vi "Priority system.vi"(0 "robot location":dbl[](array[numeric]), 1 "robot direction":string, 2 "Target distance":dbl, 3 "Display Map":dbl[][](array[numeric])) -> (7 "Map":u16[][](array[ring]), 8 "target location":dbl[](array[numeric]))   [LabVIEW 2015]
uses:
  <vilib>/robotics/Navigation/shared/WorldMap/OccupancyGridWorldMap/NI_Robotics_OccupancyGridWorldMap.lvclass
  <vilib>/robotics/Navigation/NI_Robotics_Navigation .lvlib
panel:
  out "route map":dbl[][](array[numeric])
  out "distances":dbl[](array[numeric])
  out "Indices":i32[][](array[numeric])
  out "Priority level array":dbl[][](array[numeric])
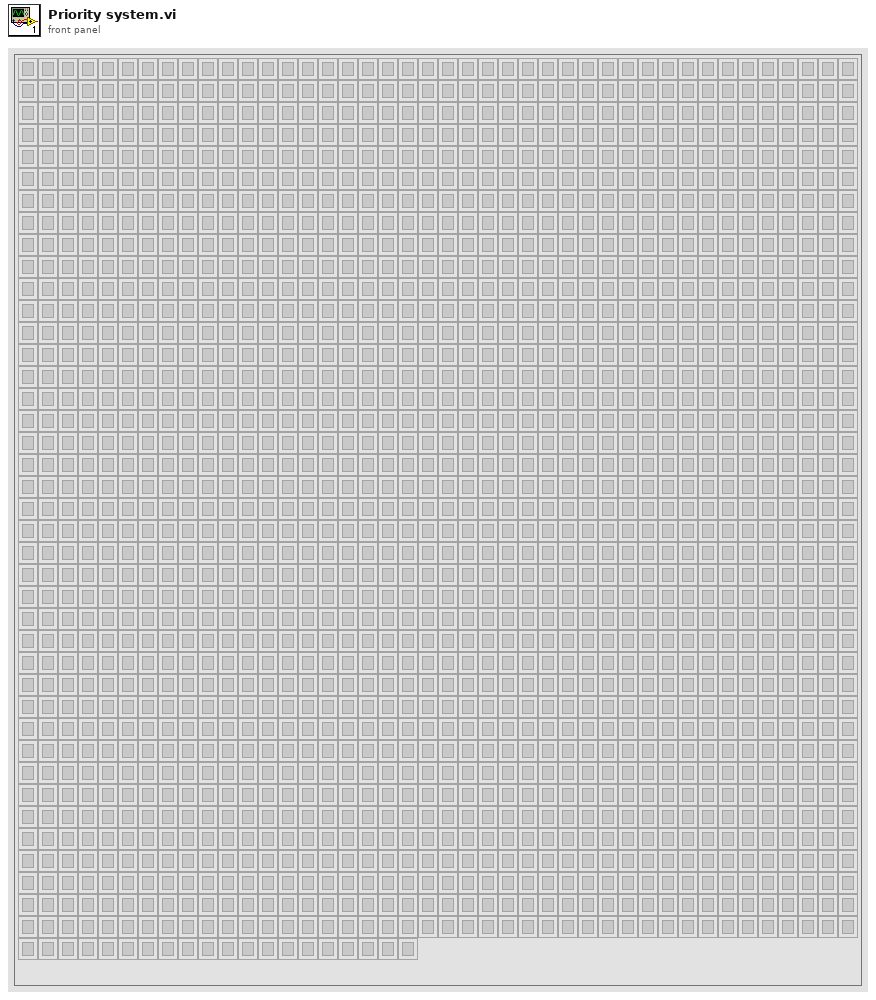
[diagram p1: front panel]
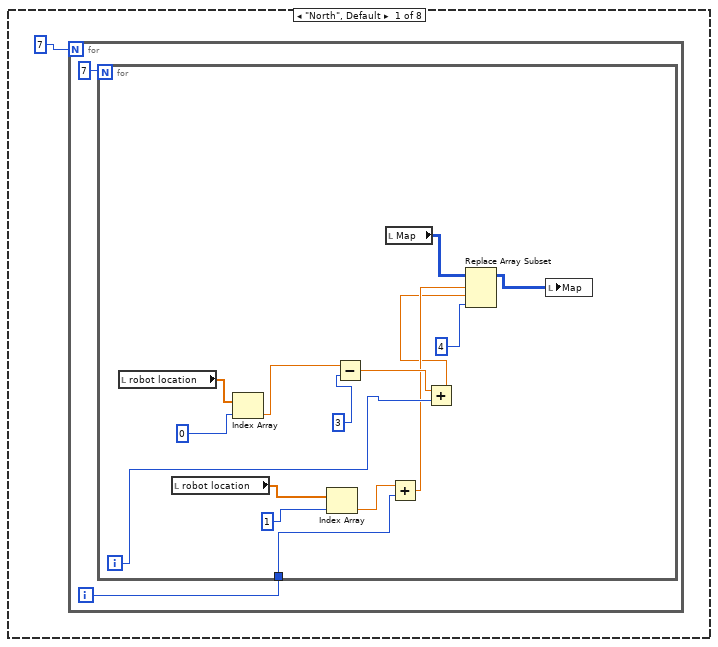
[diagram p2: hidden frame]
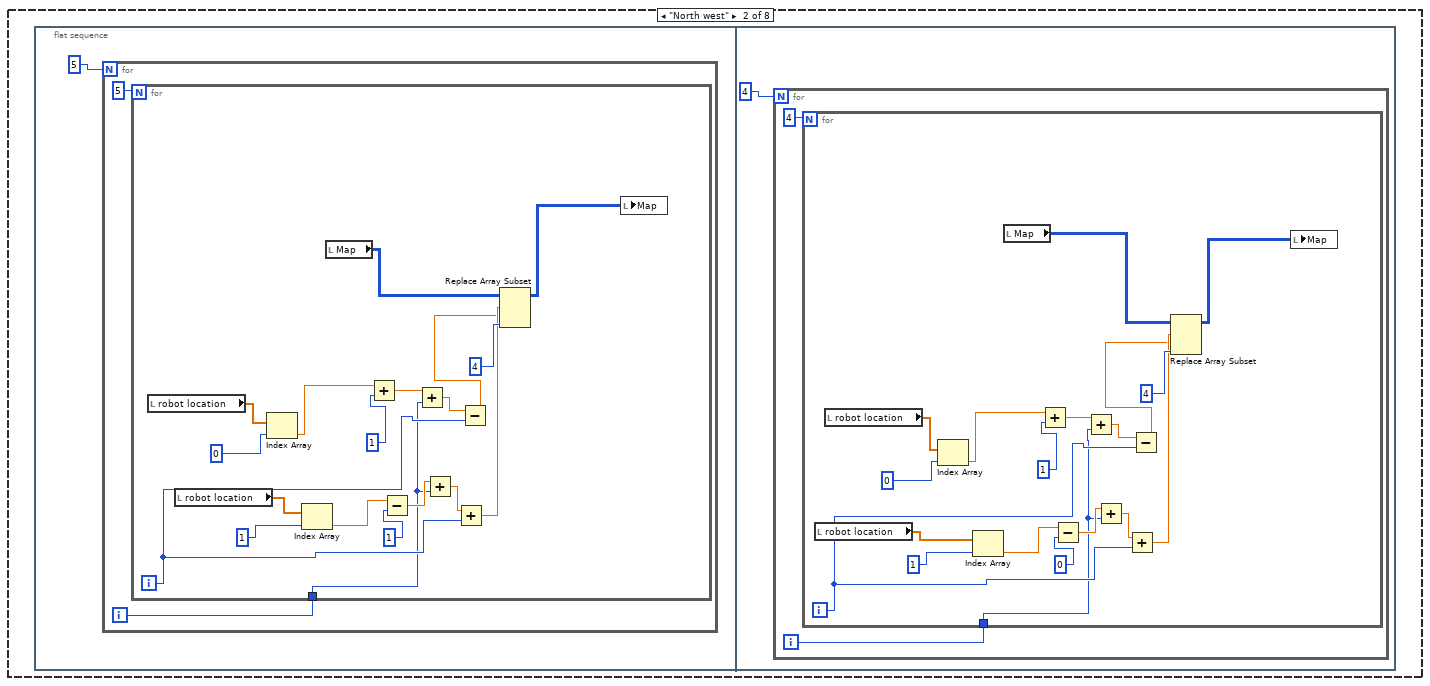
[diagram p3: hidden frame]
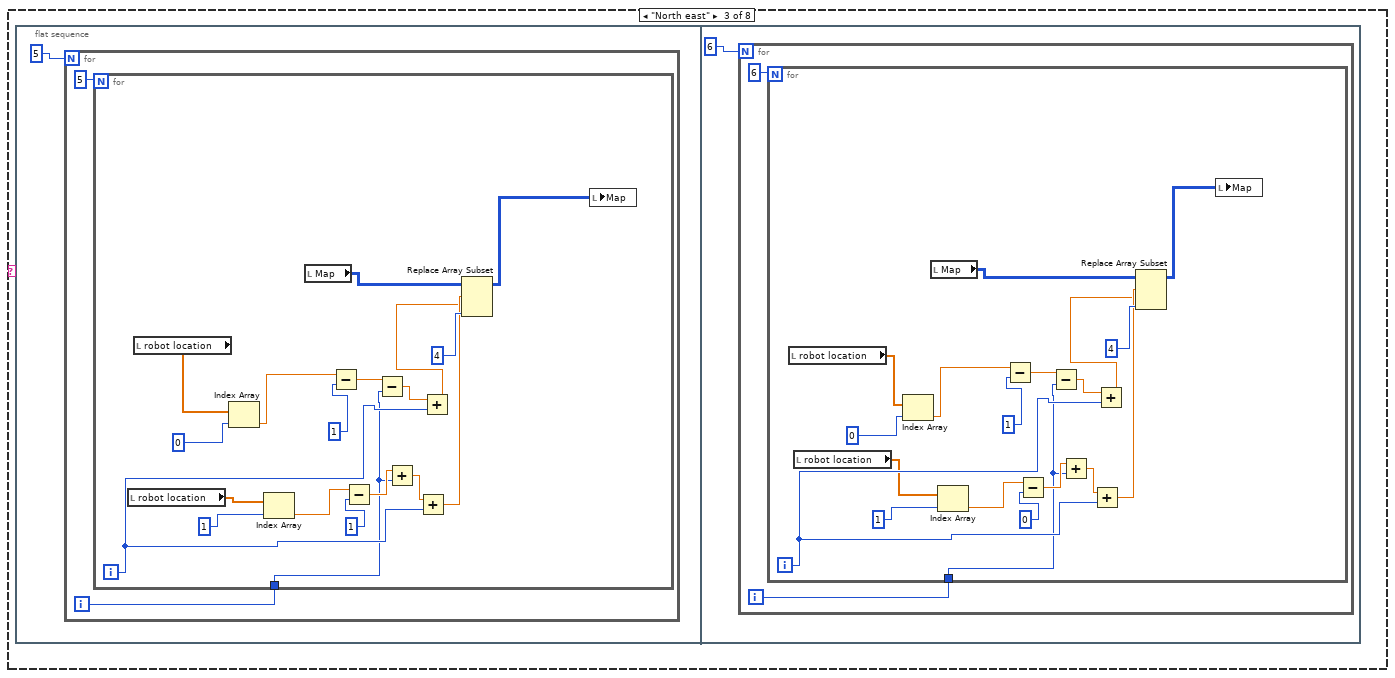
[diagram p4: hidden frame]
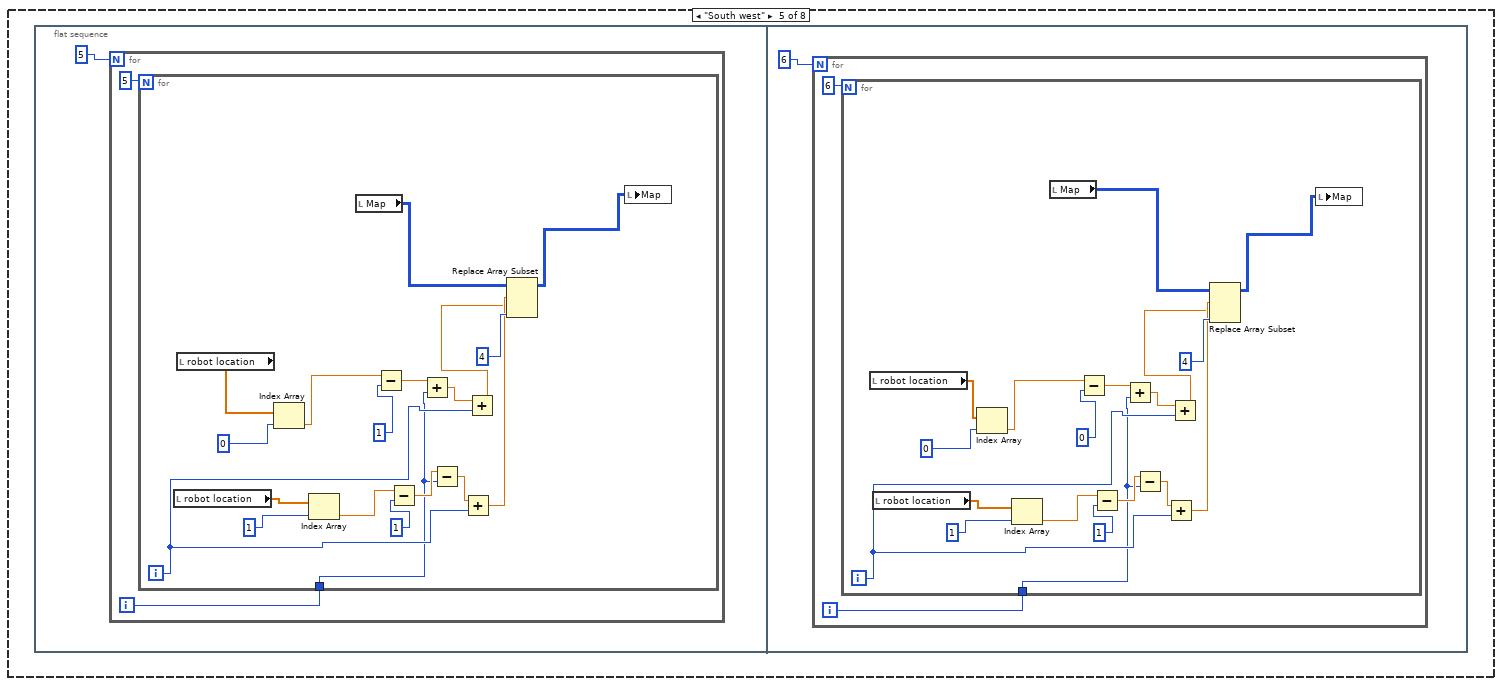
[diagram p5: hidden frame]
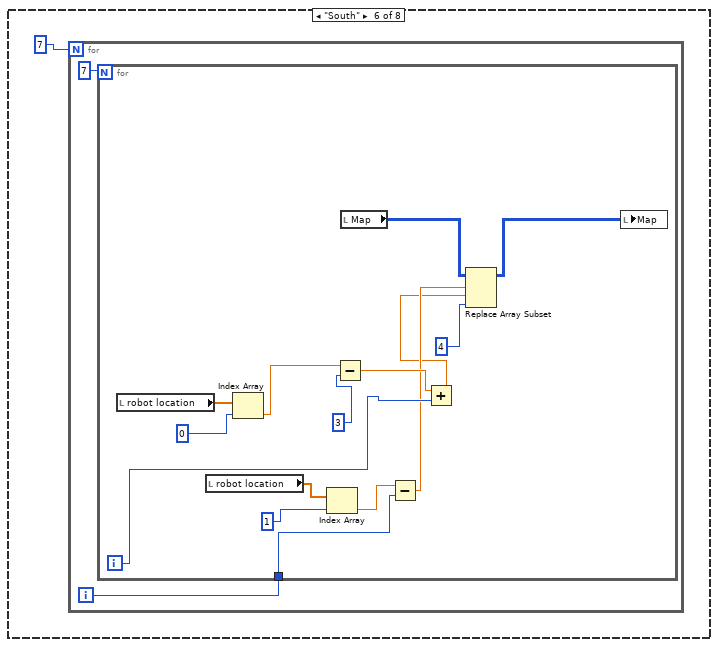
[diagram p6: hidden frame]
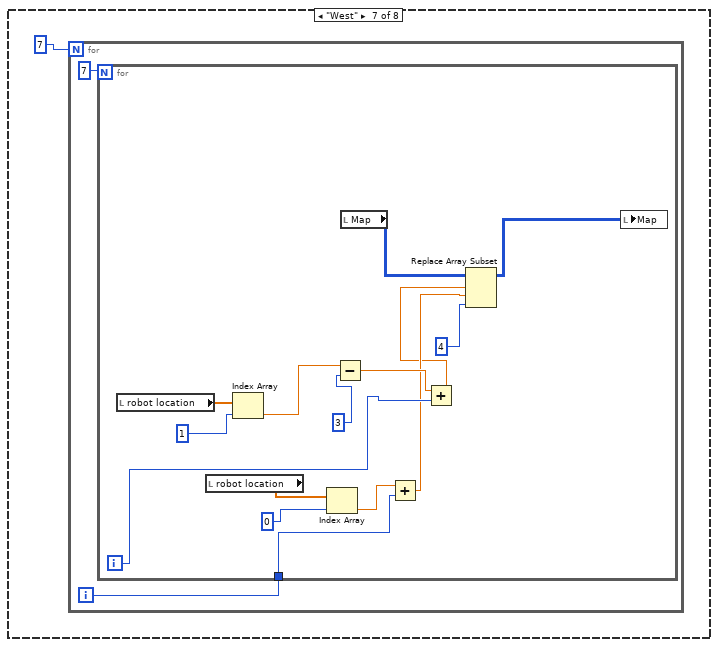
[diagram p7: hidden frame]
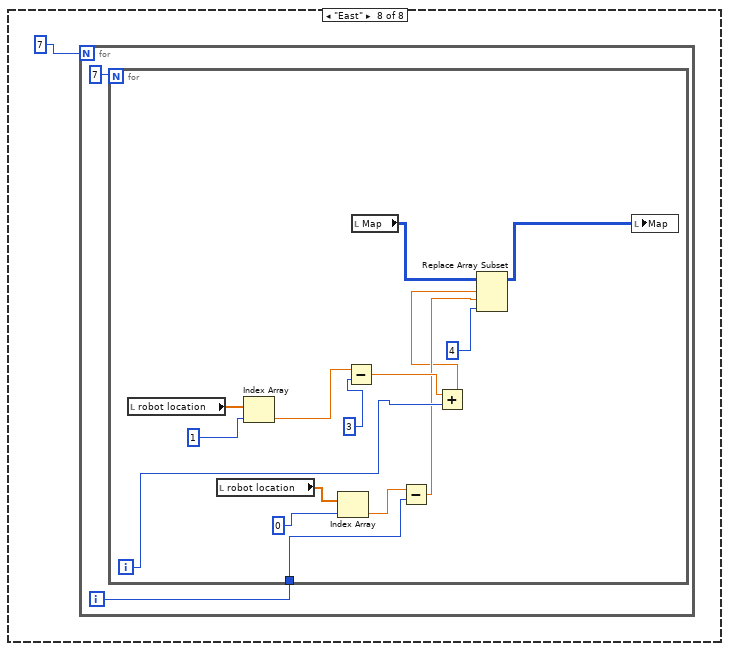
[diagram p8: hidden frame]
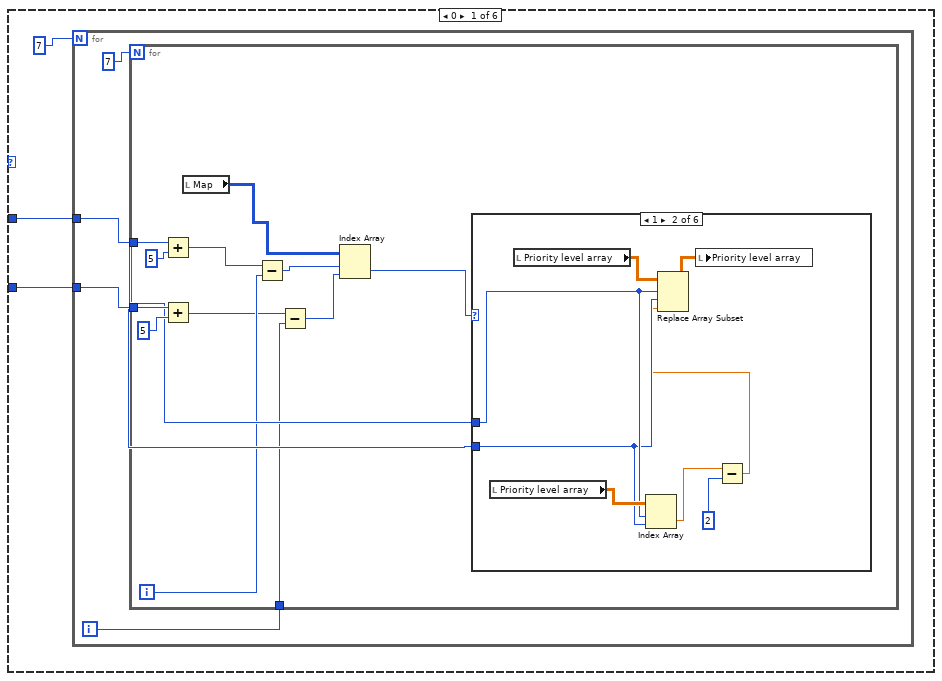
[diagram p9: hidden frame]
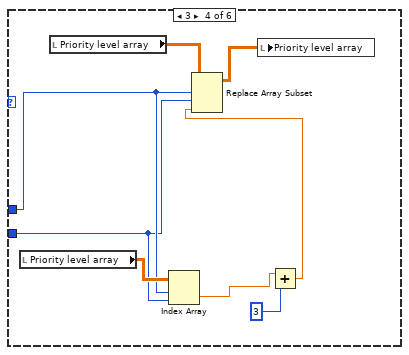
[diagram p12: hidden frame]
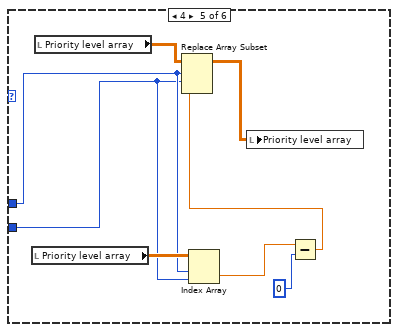
[diagram p13: hidden frame]
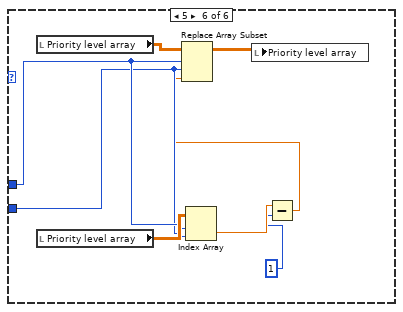
[diagram p14: hidden frame]
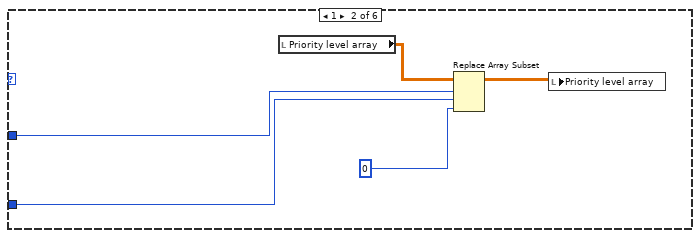
[diagram p15: hidden frame]
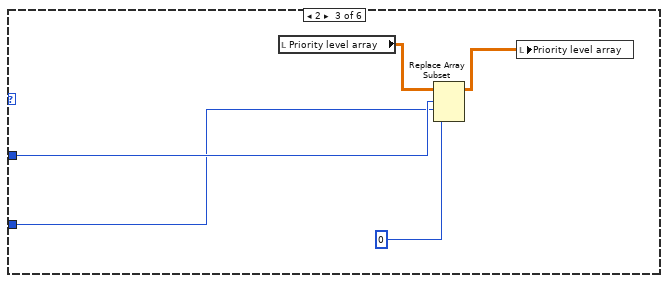
[diagram p16: hidden frame]
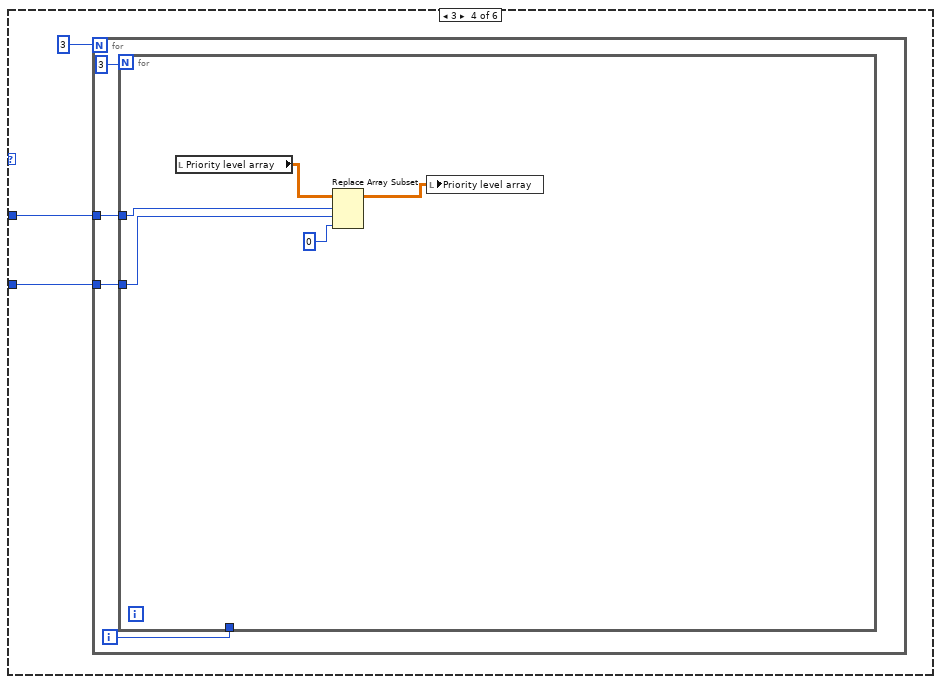
[diagram p17: hidden frame]
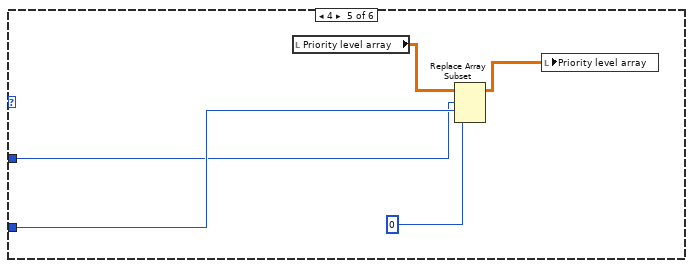
[diagram p18: hidden frame]
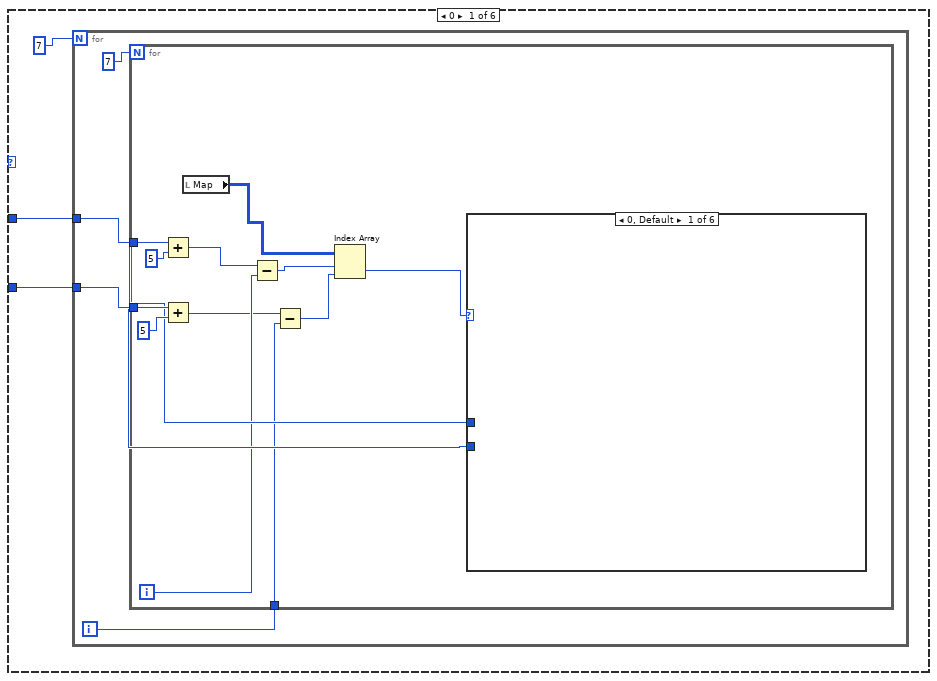
[diagram p20: hidden frame]
diagram:
  n1 = flat-sequence {
    frame #0 {
      "Map" <- "Display Map"
      "Priority level array" <- "Display Map"
      "route map" <- "Display Map"
    }
    frame #1 {
      n2 = for {
        N: 40 -> [_]
        i -> [w3]
        n3 = for {
          N: 40 -> [_]
          tunnel: w3 -> [w9]
          i -> [w10]
          n4 = local read "Priority level array"() -> (w5:dbl[][])
          n5 = local read "route map"() -> (w6:dbl[][])
          n6 = Replace Array Subset(array=w6, new element=0, index (row)=w10, index (col)=w9) -> (w11:dbl[][])
          n7 = Replace Array Subset(array=w5, new element=15, index (row)=w10, index (col)=w9) -> (w12:dbl[][])
          n8 = local write "Priority level array"(w12) -> ()
          n9 = local write "route map"(w11) -> ()
        }
      }
    }
    frame #2 {
      n10 = case shown="\"South east\"" "robot direction" {
        frame "North", Default {
          n11 = for {
            N: 7 -> [_]
            i -> [w15]
            n12 = for {
              N: 7 -> [_]
              tunnel: w15 -> [w23]
              i -> [w27]
              n13 = local read "robot location"() -> (w18:dbl[])
              n14 = local read "robot location"() -> (w17:dbl[])
              n15 = Index Array(array=w18, index=0) -> (element=w20:dbl)
              n16 = Index Array(array=w17, index=1) -> (element=w19:dbl)
              n17 = Subtract(x=w20, y=3) -> (x-y=w26:dbl)
              n18 = local read "Map"() -> (w22:u16[][])
              n19 = Add(x=w19, y=w23) -> (x+y=w25:dbl)
              n20 = Add(x=w26, y=w27) -> (x+y=w24:dbl)
              n21 = Replace Array Subset(array=w22, new element=4, index (row)=w25, index (col)=w24) -> (w21:u16[][])
              n22 = local write "Map"(w21) -> ()
            }
          }
        }
        frame "North west" {
          n23 = flat-sequence {
            frame #0 {
              n24 = for {
                N: 5 -> [_]
                i -> [w33]
                n25 = for {
                  N: 5 -> [_]
                  tunnel: w33 -> [w35]
                  i -> [w46]
                  n26 = local read "robot location"() -> (w41:dbl[])
                  n27 = local read "robot location"() -> (w40:dbl[])
                  n28 = Index Array(array=w41, index=0) -> (element=w47:dbl)
                  n29 = Index Array(array=w40, index=1) -> (element=w45:dbl)
                  n30 = local read "Map"() -> (w39:u16[][])
                  n31 = Add(x=w47, y=1) -> (x+y=w37:dbl)
                  n32 = Subtract(x=w45, y=1) -> (x-y=w43:dbl)
                  n33 = Add(x=w37, y=w35) -> (x+y=w36:dbl)
                  n34 = Add(x=w43, y=w35) -> (x+y=w42:dbl)
                  n35 = Add(x=w42, y=w46) -> (x+y=w49:dbl)
                  n36 = Subtract(x=w36, y=w46) -> (x-y=w48:dbl)
                  n37 = Replace Array Subset(array=w39, new element=4, index (row)=w49, index (col)=w48) -> (w38:u16[][])
                  n38 = local write "Map"(w38) -> ()
                }
              }
            }
            frame #1 {
              n39 = for {
                N: 4 -> [_]
                i -> [w55]
                n40 = for {
                  N: 4 -> [_]
                  tunnel: w55 -> [w62]
                  i -> [w68]
                  n41 = local read "robot location"() -> (w57:dbl[])
                  n42 = local read "robot location"() -> (w58:dbl[])
                  n43 = Index Array(array=w58, index=0) -> (element=w69:dbl)
                  n44 = Index Array(array=w57, index=1) -> (element=w67:dbl)
                  n45 = local read "Map"() -> (w60:u16[][])
                  n46 = Add(x=w69, y=1) -> (x+y=w65:dbl)
                  n47 = Subtract(x=w67, y=0) -> (x-y=w64:dbl)
                  n48 = Add(x=w65, y=w62) -> (x+y=w63:dbl)
                  n49 = Add(x=w64, y=w62) -> (x+y=w61:dbl)
                  n50 = Add(x=w61, y=w68) -> (x+y=w71:dbl)
                  n51 = Subtract(x=w63, y=w68) -> (x-y=w70:dbl)
                  n52 = Replace Array Subset(array=w60, new element=4, index (row)=w71, index (col)=w70) -> (w59:u16[][])
                  n53 = local write "Map"(w59) -> ()
                }
              }
            }
          }
        }
        frame "North east" {
          n54 = flat-sequence {
            frame #0 {
              n55 = for {
                N: 5 -> [_]
                i -> [w77]
                n56 = for {
                  N: 5 -> [_]
                  tunnel: w77 -> [w84]
                  i -> [w90]
                  n57 = local read "robot location"() -> (w79:dbl[])
                  n58 = local read "robot location"() -> (w80:dbl[])
                  n59 = Index Array(array=w80, index=0) -> (element=w91:dbl)
                  n60 = Index Array(array=w79, index=1) -> (element=w89:dbl)
                  n61 = local read "Map"() -> (w81:u16[][])
                  n62 = Subtract(x=w91, y=1) -> (x-y=w87:dbl)
                  n63 = Subtract(x=w89, y=1) -> (x-y=w86:dbl)
                  n64 = Subtract(x=w87, y=w84) -> (x-y=w85:dbl)
                  n65 = Add(x=w86, y=w84) -> (x+y=w83:dbl)
                  n66 = Add(x=w83, y=w90) -> (x+y=w93:dbl)
                  n67 = Add(x=w85, y=w90) -> (x+y=w92:dbl)
                  n68 = Replace Array Subset(array=w81, new element=4, index (row)=w93, index (col)=w92) -> (w82:u16[][])
                  n69 = local write "Map"(w82) -> ()
                }
              }
            }
            frame #1 {
              n70 = for {
                N: 6 -> [_]
                i -> [w99]
                n71 = for {
                  N: 6 -> [_]
                  tunnel: w99 -> [w101]
                  i -> [w112]
                  n72 = local read "robot location"() -> (w103:dbl[])
                  n73 = local read "robot location"() -> (w102:dbl[])
                  n74 = Index Array(array=w103, index=0) -> (element=w113:dbl)
                  n75 = local read "Map"() -> (w105:u16[][])
                  n76 = Index Array(array=w102, index=1) -> (element=w111:dbl)
                  n77 = Subtract(x=w113, y=1) -> (x-y=w109:dbl)
                  n78 = Subtract(x=w111, y=0) -> (x-y=w108:dbl)
                  n79 = Subtract(x=w109, y=w101) -> (x-y=w107:dbl)
                  n80 = Add(x=w108, y=w101) -> (x+y=w106:dbl)
                  n81 = Add(x=w106, y=w112) -> (x+y=w115:dbl)
                  n82 = Add(x=w107, y=w112) -> (x+y=w114:dbl)
                  n83 = Replace Array Subset(array=w105, new element=4, index (row)=w115, index (col)=w114) -> (w104:u16[][])
                  n84 = local write "Map"(w104) -> ()
                }
              }
            }
          }
        }
        frame "South east" {
          n85 = flat-sequence {
            frame #0 {
              n86 = for {
                N: 5 -> [_]
                i -> [w121]
                n87 = for {
                  N: 5 -> [_]
                  tunnel: w121 -> [w129]
                  i -> [w123]
                  n88 = local read "robot location"() -> (w125:dbl[])
                  n89 = local read "robot location"() -> (w124:dbl[])
                  n90 = Index Array(array=w125, index=0) -> (element=w135:dbl)
                  n91 = Index Array(array=w124, index=1) -> (element=w134:dbl)
                  n92 = Add(x=w135, y=1) -> (x+y=w132:dbl)
                  n93 = local read "Map"() -> (w126:u16[][])
                  n94 = Subtract(x=w134, y=1) -> (x-y=w131:dbl)
                  n95 = Subtract(x=w132, y=w129) -> (x-y=w130:dbl)
                  n96 = Add(x=w131, y=w129) -> (x+y=w128:dbl)
                  n97 = Subtract(x=w128, y=w123) -> (x-y=w137:dbl)
                  n98 = Subtract(x=w130, y=w123) -> (x-y=w136:dbl)
                  n99 = Replace Array Subset(array=w126, new element=4, index (row)=w137, index (col)=w136) -> (w127:u16[][])
                  n100 = local write "Map"(w127) -> ()
                }
              }
            }
            frame #1 {
              n101 = for {
                N: 4 -> [_]
                i -> [w143]
                n102 = for {
                  N: 4 -> [_]
                  tunnel: w143 -> [w151]
                  i -> [w148]
                  n103 = local read "robot location"() -> (w149:dbl[])
                  n104 = local read "robot location"() -> (w147:dbl[])
                  n105 = Index Array(array=w149, index=0) -> (element=w157:dbl)
                  n106 = Index Array(array=w147, index=1) -> (element=w156:dbl)
                  n107 = Add(x=w157, y=0) -> (x+y=w154:dbl)
                  n108 = local read "Map"() -> (w146:u16[][])
                  n109 = Subtract(x=w156, y=1) -> (x-y=w153:dbl)
                  n110 = Subtract(x=w154, y=w151) -> (x-y=w152:dbl)
                  n111 = Add(x=w153, y=w151) -> (x+y=w150:dbl)
                  n112 = Subtract(x=w150, y=w148) -> (x-y=w159:dbl)
                  n113 = Subtract(x=w152, y=w148) -> (x-y=w158:dbl)
                  n114 = Replace Array Subset(array=w146, new element=4, index (row)=w159, index (col)=w158) -> (w145:u16[][])
                  n115 = local write "Map"(w145) -> ()
                }
              }
            }
          }
        }
        frame "South west" {
          n116 = flat-sequence {
            frame #0 {
              n117 = for {
                N: 5 -> [_]
                i -> [w165]
                n118 = for {
                  N: 5 -> [_]
                  tunnel: w165 -> [w173]
                  i -> [w179]
                  n119 = local read "robot location"() -> (w168:dbl[])
                  n120 = local read "robot location"() -> (w169:dbl[])
                  n121 = Index Array(array=w169, index=0) -> (element=w167:dbl)
                  n122 = Index Array(array=w168, index=1) -> (element=w178:dbl)
                  n123 = local read "Map"() -> (w170:u16[][])
                  n124 = Subtract(x=w167, y=1) -> (x-y=w176:dbl)
                  n125 = Subtract(x=w178, y=1) -> (x-y=w175:dbl)
                  n126 = Add(x=w176, y=w173) -> (x+y=w174:dbl)
                  n127 = Subtract(x=w175, y=w173) -> (x-y=w172:dbl)
                  n128 = Add(x=w172, y=w179) -> (x+y=w181:dbl)
                  n129 = Add(x=w174, y=w179) -> (x+y=w180:dbl)
                  n130 = Replace Array Subset(array=w170, new element=4, index (row)=w181, index (col)=w180) -> (w171:u16[][])
                  n131 = local write "Map"(w171) -> ()
                }
              }
            }
            frame #1 {
              n132 = for {
                N: 6 -> [_]
                i -> [w187]
                n133 = for {
                  N: 6 -> [_]
                  tunnel: w187 -> [w194]
                  i -> [w200]
                  n134 = local read "robot location"() -> (w190:dbl[])
                  n135 = local read "robot location"() -> (w189:dbl[])
                  n136 = Index Array(array=w190, index=0) -> (element=w201:dbl)
                  n137 = Index Array(array=w189, index=1) -> (element=w199:dbl)
                  n138 = local read "Map"() -> (w192:u16[][])
                  n139 = Subtract(x=w201, y=0) -> (x-y=w197:dbl)
                  n140 = Subtract(x=w199, y=1) -> (x-y=w196:dbl)
                  n141 = Add(x=w197, y=w194) -> (x+y=w195:dbl)
                  n142 = Subtract(x=w196, y=w194) -> (x-y=w193:dbl)
                  n143 = Add(x=w193, y=w200) -> (x+y=w203:dbl)
                  n144 = Add(x=w195, y=w200) -> (x+y=w202:dbl)
                  n145 = Replace Array Subset(array=w192, new element=4, index (row)=w203, index (col)=w202) -> (w191:u16[][])
                  n146 = local write "Map"(w191) -> ()
                }
              }
            }
          }
        }
        frame "South" {
          n147 = for {
            N: 7 -> [_]
            i -> [w209]
            n148 = for {
              N: 7 -> [_]
              tunnel: w209 -> [w217]
              i -> [w221]
              n149 = local read "robot location"() -> (w214:dbl[])
              n150 = local read "robot location"() -> (w213:dbl[])
              n151 = Index Array(array=w214, index=0) -> (element=w212:dbl)
              n152 = Index Array(array=w213, index=1) -> (element=w211:dbl)
              n153 = Subtract(x=w212, y=3) -> (x-y=w220:dbl)
              n154 = local read "Map"() -> (w216:u16[][])
              n155 = Subtract(x=w211, y=w217) -> (x-y=w219:dbl)
              n156 = Add(x=w220, y=w221) -> (x+y=w218:dbl)
              n157 = Replace Array Subset(array=w216, new element=4, index (row)=w219, index (col)=w218) -> (w215:u16[][])
              n158 = local write "Map"(w215) -> ()
            }
          }
        }
        frame "West" {
          n159 = for {
            N: 7 -> [_]
            i -> [w227]
            n160 = for {
              N: 7 -> [_]
              tunnel: w227 -> [w237]
              i -> [w239]
              n161 = local read "robot location"() -> (w232:dbl[])
              n162 = local read "robot location"() -> (w231:dbl[])
              n163 = Index Array(array=w232, index=1) -> (element=w230:dbl)
              n164 = Index Array(array=w231, index=0) -> (element=w229:dbl)
              n165 = Subtract(x=w230, y=3) -> (x-y=w238:dbl)
              n166 = local read "Map"() -> (w234:u16[][])
              n167 = Add(x=w229, y=w237) -> (x+y=w236:dbl)
              n168 = Add(x=w238, y=w239) -> (x+y=w235:dbl)
              n169 = Replace Array Subset(array=w234, new element=4, index (row)=w235, index (col)=w236) -> (w233:u16[][])
              n170 = local write "Map"(w233) -> ()
            }
          }
        }
        frame "East" {
          n171 = for {
            N: 7 -> [_]
            i -> [w245]
            n172 = for {
              N: 7 -> [_]
              tunnel: w245 -> [w249]
              i -> [w251]
              n173 = local read "robot location"() -> (w258:dbl[])
              n174 = local read "robot location"() -> (w256:dbl[])
              n175 = Index Array(array=w258, index=1) -> (element=w253:dbl)
              n176 = Index Array(array=w256, index=0) -> (element=w254:dbl)
              n177 = Subtract(x=w253, y=3) -> (x-y=w250:dbl)
              n178 = local read "Map"() -> (w261:u16[][])
              n179 = Subtract(x=w254, y=w249) -> (x-y=w248:dbl)
              n180 = Add(x=w250, y=w251) -> (x+y=w247:dbl)
              n181 = Replace Array Subset(array=w261, new element=4, index (row)=w247, index (col)=w248) -> (w260:u16[][])
              n182 = local write "Map"(w260) -> ()
            }
          }
        }
      }
    }
    frame #3 {
      n183 = local read "robot location"() -> (w267:dbl[])
      n184 = Divide(x="Target distance", y=50.0) -> (x/y=w269:dbl)
      n185 = Index Array(array=w267, index #1=0, index #2=1) -> (element #1=w264:dbl, element #2=w262:dbl)
      n186 = Round To Nearest(number=w269) -> (nearest integer value=w263:dbl)
      n187 = for {
        N: 3 -> [_]
        tunnel: w264 -> [w274]
        tunnel: w263 -> [w273]
        tunnel: w262 -> [w272]
        i -> [w276]
        n188 = for {
          N: 3 -> [_]
          tunnel: w276 -> [w281]
          tunnel: w274 -> [w277]
          tunnel: w273 -> [w279]
          tunnel: w272 -> [w280]
          i -> [w285]
          n189 = Subtract(x=w280, y=w279) -> (x-y=w278:dbl)
          n190 = Subtract(x=w278, y=1) -> (x-y=w287:dbl)
          n191 = Add(x=w287, y=w285) -> (x+y=w286:dbl)
          n192 = Subtract(x=w277, y=1) -> (x-y=w284:dbl)
          n193 = local read "Map"() -> (w291:u16[][])
          n194 = Add(x=w284, y=w281) -> (x+y=w283:dbl)
          n195 = Replace Array Subset(array=w291, new element=1, index (row)=w286, index (col)=w283) -> (w290:u16[][])
          n196 = local write "Map"(w290) -> ()
        }
      }
    }
    frame #4 {
      n197 = for {
        N: 40 -> [_]
        i -> [w293]
        n198 = for {
          N: 40 -> [_]
          tunnel: w293 -> [w297]
          i -> [w296]
          n199 = local read "Map"() -> (w298:u16[][])
          n200 = Index Array(array=w298, index (row)=w296, index (col)=w297) -> (element=w295:u16)
          n201 = case shown="5, Default" w295 {
            tunnel: w297 -> [w301 w351 w357 w362 w374 w378]
            tunnel: w296 -> [w300 w350 w358 w361 w373 w379]
            frame 0 {
              n202 = for {
                N: 7 -> [_]
                tunnel: w301 -> [w305]
                tunnel: w300 -> [w304]
                i -> [w302]
                n203 = for {
                  N: 7 -> [_]
                  tunnel: w305 -> [w314]
                  tunnel: w304 -> [w313]
                  tunnel: w302 -> [w309]
                  i -> [w311]
                  n204 = Add(x=w313, y=5) -> (x+y=w312:i32)
                  n205 = Add(x=w314, y=5) -> (x+y=w310:i32)
                  n206 = local read "Map"() -> (w317:u16[][])
                  n207 = Subtract(x=w312, y=w311) -> (x-y=w307:i32)
                  n208 = Subtract(x=w310, y=w309) -> (x-y=w308:i32)
                  n209 = Index Array(array=w317, index (row)=w307, index (col)=w308) -> (element=w306:u16)
                  n210 = case shown="1" w306 {
                    tunnel: w314 -> [_ w321 _ w330 w337 w345]
                    tunnel: w313 -> [_ w322 _ w331 w338 w346]
                    frame 0, Default {
                    }
                    frame 1 {
                      n211 = local read "Priority level array"() -> (w325:dbl[][])
                      n212 = local read "Priority level array"() -> (w324:dbl[][])
                      n213 = Index Array(array=w325, index (row)=w322, index (col)=w321) -> (element=w320:dbl)
                      n214 = Subtract(x=w320, y=2) -> (x-y=w318:dbl)
                      n215 = Replace Array Subset(array=w324, new element=w318, index (row)=w322, index (col)=w321) -> (w323:dbl[][])
                      n216 = local write "Priority level array"(w323) -> ()
                    }
                    frame 2 {
                    }
                    frame 3 {
                      n217 = local read "Priority level array"() -> (w332:dbl[][])
                      n218 = local read "Priority level array"() -> (w333:dbl[][])
                      n219 = Index Array(array=w332, index (row)=w331, index (col)=w330) -> (element=w329:dbl)
                      n220 = Add(x=w329, y=3) -> (x+y=w327:dbl)
                      n221 = Replace Array Subset(array=w333, new element=w327, index (row)=w331, index (col)=w330) -> (w328:dbl[][])
                      n222 = local write "Priority level array"(w328) -> ()
                    }
                    frame 4 {
                      n223 = local read "Priority level array"() -> (w339:dbl[][])
                      n224 = local read "Priority level array"() -> (w341:dbl[][])
                      n225 = Index Array(array=w339, index (row)=w338, index (col)=w337) -> (element=w336:dbl)
                      n226 = Subtract(x=w336, y=0) -> (x-y=w335:dbl)
                      n227 = Replace Array Subset(array=w341, new element=w335, index (row)=w338, index (col)=w337) -> (w340:dbl[][])
                      n228 = local write "Priority level array"(w340) -> ()
                    }
                    frame 5 {
                      n229 = local read "Priority level array"() -> (w347:dbl[][])
                      n230 = local read "Priority level array"() -> (w349:dbl[][])
                      n231 = Index Array(array=w349, index (row)=w346, index (col)=w345) -> (element=w344:dbl)
                      n232 = Subtract(x=w344, y=1) -> (x-y=w343:dbl)
                      n233 = Replace Array Subset(array=w347, new element=w343, index (row)=w346, index (col)=w345) -> (w348:dbl[][])
                      n234 = local write "Priority level array"(w348) -> ()
                    }
                  }
                }
              }
            }
            frame 1 {
              n235 = local read "Priority level array"() -> (w354:dbl[][])
              n236 = Replace Array Subset(array=w354, new element=0, index (row)=w350, index (col)=w351) -> (w353:dbl[][])
              n237 = local write "Priority level array"(w353) -> ()
            }
            frame 2 {
              n238 = local read "Priority level array"() -> (w359:dbl[][])
              n239 = Replace Array Subset(array=w359, new element=0, index (row)=w358, index (col)=w357) -> (w356:dbl[][])
              n240 = local write "Priority level array"(w356) -> ()
            }
            frame 3 {
              n241 = for {
                N: 3 -> [_]
                tunnel: w362 -> [w366]
                tunnel: w361 -> [w365]
                i -> [w363]
                n242 = for {
                  N: 3 -> [_]
                  tunnel: w366 -> [w367]
                  tunnel: w365 -> [w368]
                  tunnel: w363 -> [_]
                  n243 = local read "Priority level array"() -> (w371:dbl[][])
                  n244 = Replace Array Subset(array=w371, new element=0, index (row)=w368, index (col)=w367) -> (w370:dbl[][])
                  n245 = local write "Priority level array"(w370) -> ()
                }
              }
            }
            frame 4 {
              n246 = local read "Priority level array"() -> (w376:dbl[][])
              n247 = Replace Array Subset(array=w376, new element=0, index (row)=w373, index (col)=w374) -> (w375:dbl[][])
              n248 = local write "Priority level array"(w375) -> ()
            }
            frame 5, Default {
              n249 = local read "Priority level array"() -> (w381:dbl[][])
              n250 = Replace Array Subset(array=w381, new element=0, index (row)=w379, index (col)=w378) -> (w380:dbl[][])
              n251 = local write "Priority level array"(w380) -> ()
            }
          }
        }
      }
    }
    frame #5 {
      n252 = local read "Priority level array"() -> (w383:dbl[][])
      n253 = for {
        tunnel: [w386] -> _ mode=indexing
        shift-right: [w390] -> w385
        shift-left: i32[][] [] -> [w388]
        tunnel: w383 -> [w386] mode=indexing
        i -> [w392]
        n254 = Increment(x=w392) -> (x+1=w391:i32)
        n255 = for {
          tunnel: w386 -> [w401] mode=indexing
          tunnel: w391 -> [w397]
          shift-right: [w396] -> w389
          shift-left: i32[][] [] -> [w395]
          i -> [w399]
          n256 = local read "Priority level array"() -> (w394:dbl[][])
          n257 = Array Max & Min(array=w394) -> (max value=w393:dbl)  [unwired: 3 out]
          n258 = Equal?(x=w401, y=w393) -> (x = y?=w400:bool)
          n259 = Increment(x=w399) -> (x+1=w398:i32)
          n260 = case shown="True" w400 {
            tunnel: w398 -> [_ w407]
            tunnel: w397 -> [_ w406]
            tunnel: [w402 w404] -> w396
            tunnel: w395 -> [w402 w403]
            frame False {
            }
            frame True {
              n261 = Build Array(w407, w406) -> (w405:i32[])
              n262 = Build Array (concatenate)(w403, w405) -> (w404:i32[][])
            }
          }
        }
        n263 = Build Array (concatenate)(w388, w389) -> (w390:i32[][])
      }
      "Indices" <- w385
      "distances" <- i32[] [0, 0, 0, 0, 0, 0, 0, 0, 0, 0]
    }
    frame #6 {
      n264 = for {
        N: 10 -> [_]
        i -> [w411]
        n265 = local read "Indices"() -> (w432:i32[][])
        n266 = Index Array(array=w432, index (row)=w411, index (col)=0) -> (element=w425:i32)
        n267 = Index Array(array=w432, index (row)=w411, index (col)=1) -> (element=w424:i32)
        n268 = Index Array(array="robot location", index=1) -> (element=w427:dbl)
        n269 = Index Array(array="robot location", index=0) -> (element=w429:dbl)
        n270 = Add(x=w427, y=1) -> (x+y=w422:dbl)
        n271 = Add(x=w429, y=1) -> (x+y=w423:dbl)
        n272 = Subtract(x=w425, y=w423) -> (x-y=w421:dbl)
        n273 = Subtract(x=w424, y=w422) -> (x-y=w414:dbl)
        n274 = Square(x=w414) -> (x^2=w420:dbl)
        n275 = Square(x=w421) -> (x^2=w419:dbl)
        n276 = Add(x=w419, y=w420) -> (x+y=w418:dbl)
        n277 = local read "distances"() -> (w417:dbl[])
        n278 = Square Root(x=w418) -> (sqrt(x)=w415:dbl)
        n279 = Replace Array Subset(array=w417, new element=w415, index=w411) -> (w416:dbl[])
        n280 = local write "distances"(w416) -> ()
      }
      "target location" <- i32[] [0, 0]
    }
    frame #7 {
      n281 = local read "distances"() -> (w440:dbl[])
      n282 = local read "Indices"() -> (w433:i32[][])
      n283 = Array Max & Min(array=w440) -> (min index (indices)=w435:i32)  [unwired: 3 out]
      n284 = local read "target location"() -> (w437:dbl[])
      n285 = Index Array(array=w433, index (row)=w435, index (col)=0) -> (element=w438:i32)
      n286 = Replace Array Subset(array=w437, new element=w438, index=0) -> (w439:dbl[])
      n287 = local write "target location"(w439) -> ()
    }
    frame #8 {
      n288 = local read "distances"() -> (w447:dbl[])
      n289 = local read "Indices"() -> (w446:i32[][])
      n290 = Array Max & Min(array=w447) -> (min index (indices)=w448:i32)  [unwired: 3 out]
      n291 = local read "target location"() -> (w443:dbl[])
      n292 = Index Array(array=w446, index (row)=w448, index (col)=1) -> (element=w442:i32)
      n293 = Replace Array Subset(array=w443, new element=w442, index=1) -> (w441:dbl[])
      n294 = local write "target location"(w441) -> ()
    }
    frame #9 {
      n295 = local read "target location"() -> (w455:dbl[])
      n296 = Index Array(array=w455, index #1=0, index #2=1) -> (element #1=w452:dbl, element #2=w451:dbl)
      n297 = local read "Map"() -> (w458:u16[][])
      n298 = Decrement(x=w451) -> (x-1=w450:dbl)
      n299 = Decrement(x=w452) -> (x-1=w449:dbl)
      n300 = Replace Array Subset(array=w458, new element=4, index (row)=w450, index (col)=w449) -> (w457:u16[][])
      n301 = local write "Map"(w457) -> ()
    }
    frame #10 {
      n302 = for {
        N: 40 -> [_]
        i -> [w460]
        n303 = for {
          N: 40 -> [_]
          tunnel: w460 -> [w464]
          i -> [w463]
          n304 = local read "Map"() -> (w465:u16[][])
          n305 = Index Array(array=w465, index (row)=w463, index (col)=w464) -> (element=w462:u16)
          n306 = case shown="2" w462 {
            tunnel: w464 -> [w468 w518 w524 w529 w541 w545]
            tunnel: w463 -> [w467 w517 w525 w528 w540 w546]
            frame 0 {
              n307 = for {
                N: 7 -> [_]
                tunnel: w468 -> [w472]
                tunnel: w467 -> [w471]
                i -> [w469]
                n308 = for {
                  N: 7 -> [_]
                  tunnel: w472 -> [w481]
                  tunnel: w471 -> [w480]
                  tunnel: w469 -> [w476]
                  i -> [w478]
                  n309 = Add(x=w480, y=5) -> (x+y=w479:i32)
                  n310 = Add(x=w481, y=5) -> (x+y=w477:i32)
                  n311 = local read "Map"() -> (w484:u16[][])
                  n312 = Subtract(x=w479, y=w478) -> (x-y=w474:i32)
                  n313 = Subtract(x=w477, y=w476) -> (x-y=w475:i32)
                  n314 = Index Array(array=w484, index (row)=w474, index (col)=w475) -> (element=w473:u16)
                  n315 = case shown="0, Default" w473 {
                    tunnel: w481 -> [_ w488 _ w497 w504 w512]
                    tunnel: w480 -> [_ w489 _ w498 w505 w513]
                    frame 0, Default {
                    }
                    frame 1 {
                      n316 = local read "route map"() -> (w492:dbl[][])
                      n317 = local read "route map"() -> (w491:dbl[][])
                      n318 = Index Array(array=w492, index (row)=w489, index (col)=w488) -> (element=w487:dbl)
                      n319 = Add(x=w487, y=2) -> (x+y=w485:dbl)
                      n320 = Replace Array Subset(array=w491, new element=w485, index (row)=w489, index (col)=w488) -> (w490:dbl[][])
                      n321 = local write "route map"(w490) -> ()
                    }
                    frame 2 {
                    }
                    frame 3 {
                      n322 = local read "route map"() -> (w499:dbl[][])
                      n323 = local read "route map"() -> (w500:dbl[][])
                      n324 = Index Array(array=w499, index (row)=w498, index (col)=w497) -> (element=w496:dbl)
                      n325 = Add(x=w496, y=0) -> (x+y=w494:dbl)
                      n326 = Replace Array Subset(array=w500, new element=w494, index (row)=w498, index (col)=w497) -> (w495:dbl[][])
                      n327 = local write "route map"(w495) -> ()
                    }
                    frame 4 {
                      n328 = local read "route map"() -> (w506:dbl[][])
                      n329 = local read "route map"() -> (w508:dbl[][])
                      n330 = Index Array(array=w506, index (row)=w505, index (col)=w504) -> (element=w503:dbl)
                      n331 = Add(x=w503, y=1) -> (x+y=w502:dbl)
                      n332 = Replace Array Subset(array=w508, new element=w502, index (row)=w505, index (col)=w504) -> (w507:dbl[][])
                      n333 = local write "route map"(w507) -> ()
                    }
                    frame 5 {
                      n334 = local read "route map"() -> (w514:dbl[][])
                      n335 = local read "route map"() -> (w516:dbl[][])
                      n336 = Index Array(array=w516, index (row)=w513, index (col)=w512) -> (element=w511:dbl)
                      n337 = Add(x=w511, y=1) -> (x+y=w510:dbl)
                      n338 = Replace Array Subset(array=w514, new element=w510, index (row)=w513, index (col)=w512) -> (w515:dbl[][])
                      n339 = local write "route map"(w515) -> ()
                    }
                  }
                }
              }
            }
            frame 1 {
              n340 = local read "route map"() -> (w521:dbl[][])
              n341 = Replace Array Subset(array=w521, new element=100, index (row)=w517, index (col)=w518) -> (w520:dbl[][])
              n342 = local write "route map"(w520) -> ()
            }
            frame 2 {
              n343 = local read "route map"() -> (w526:dbl[][])
              n344 = Replace Array Subset(array=w526, new element=0, index (row)=w525, index (col)=w524) -> (w523:dbl[][])
              n345 = local write "route map"(w523) -> ()
            }
            frame 3 {
              n346 = for {
                N: 3 -> [_]
                tunnel: w529 -> [w533]
                tunnel: w528 -> [w532]
                i -> [w530]
                n347 = for {
                  N: 3 -> [_]
                  tunnel: w533 -> [w534]
                  tunnel: w532 -> [w535]
                  tunnel: w530 -> [_]
                  n348 = local read "route map"() -> (w538:dbl[][])
                  n349 = Replace Array Subset(array=w538, new element=25, index (row)=w535, index (col)=w534) -> (w537:dbl[][])
                  n350 = local write "route map"(w537) -> ()
                }
              }
            }
            frame 4 {
              n351 = local read "route map"() -> (w543:dbl[][])
              n352 = Replace Array Subset(array=w543, new element=50, index (row)=w540, index (col)=w541) -> (w542:dbl[][])
              n353 = local write "route map"(w542) -> ()
            }
            frame 5, Default {
              n354 = local read "route map"() -> (w548:dbl[][])
              n355 = Replace Array Subset(array=w548, new element=50, index (row)=w546, index (col)=w545) -> (w547:dbl[][])
              n356 = local write "route map"(w547) -> ()
            }
          }
        }
      }
    }
    frame #11 {
      n357 = local read "route map"() -> (w561:dbl[][])
      n358 = local read "robot location"() -> (w560:dbl[])
      n359 = Multiply(x=w561, y=99) -> (x*y=w572:dbl[][])
      n360 = Add(x=w572, y=1) -> (x+y=w570:dbl[][])
      n361 = call <vilib>:"Create Occupancy Grid Map.vi"("occupancy grid"=w570) -> ("error out"=w569:errorcluster, "map reference out"=w565:refnum<data-value>)  [unwired: 9 in]
      n362 = Index Array(array=w560, index #1=0, index #2=1) -> (element #1=w550:dbl, element #2=w549:dbl)
      n363 = local read "target location"() -> (w557:dbl[])
      n364 = call <vilib>:"Get Cell Reference.vi"("error in (no error)"=w569, "y"=w550, "x"=w549, "map reference in"=w565) -> ("error out"=w568:errorcluster, "cell reference"=w566:refnum<data-value>, "map reference out"=w578:refnum<data-value>)  [unwired: 4 in, 1 out]
      n365 = Index Array(array=w557, index #1=0, index #2=1) -> (element #1=w554:dbl, element #2=w553:dbl)
      n366 = Decrement(x=w553) -> (x-1=w551:dbl)
      n367 = Decrement(x=w554) -> (x-1=w552:dbl)
      n368 = call <vilib>:"Get Cell Reference.vi"("error in (no error)"=w568, "y"=w552, "x"=w551, "map reference in"=w578) -> ("error out"=w567:errorcluster, "cell reference"=w564:refnum<data-value>, "map reference out"=w576:refnum<data-value>)  [unwired: 4 in, 1 out]
      n369 = call <vilib>:"A Star Plan.vi"("goal reference"=w564, "start reference"=w566, "map reference in"=w576) -> ("path references"=w577:refnum<data-value>[])  [unwired: 5 in, 3 out]
      n370 = call <vilib>:"Get Cells in Path.vi"("error in (no error)"=w567, "path references"=w577, "map reference in"=w576) -> ("error out"=w562:errorcluster, "y coordinates"=w575:i32[], "x coordinates"=w574:i32[], "map reference out"=w563:refnum<data-value>)  [unwired: 5 in]
      n371 = for {
        tunnel: w575 -> [w582] mode=indexing
        tunnel: w574 -> [w583] mode=indexing
        n372 = local read "Map"() -> (w579:u16[][])
        n373 = Replace Array Subset(array=w579, new element=2, index (row)=w583, index (col)=w582) -> (w580:u16[][])
        n374 = local write "Map"(w580) -> ()
      }
      n375 = call <vilib>:"Close Occupancy Grid Map.vi"("error in (no error)"=w562, "map reference in"=w563) -> ()  [unwired: 9 in, 1 out]
    }
    frame #12 {
      n376 = local read "robot location"() -> (w586:dbl[])
      n377 = local read "robot location"() -> (w587:dbl[])
      n378 = local read "Map"() -> (w588:u16[][])
      n379 = Index Array(array=w586, index=0) -> (element=w585:dbl)
      n380 = Index Array(array=w587, index=1) -> (element=w590:dbl)
      n381 = Replace Array Subset(array=w588, new element=5, index (row)=w590, index (col)=w585) -> (w589:u16[][])
      n382 = local write "Map"(w589) -> ()
    }
  }
